vi "stopVILV2G.vi"(10 "Mode":enum16{"Init", "Get", "Set"}(ring), 11 "Stop IN":bool) -> (2 "Skipped?":bool=TRUE, 3 "Stop OUT":bool)   [LabVIEW 2010]
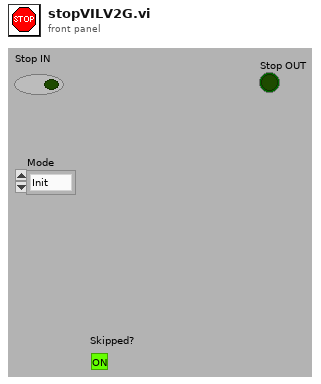
[diagram p1: front panel]
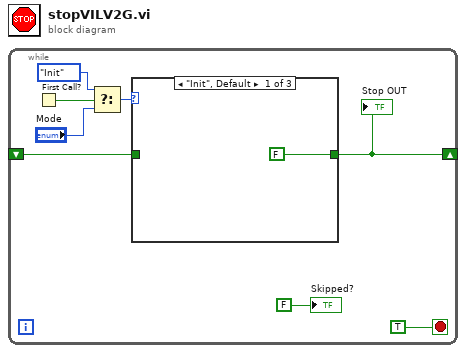
[diagram p0: block diagram]
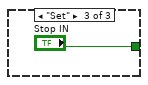
[diagram p3: hidden frame]
diagram:
  n1 = while {
    shift-right: [w6] -> _
    shift-left: _ -> [w5]
    stop <- TRUE stop-if-true
    n2 = First Call?() -> (First Call?: T/F=w3:bool)
    n3 = Select(t=enum16{"Init", "Get", "Set"}."Init" ("Mode"), s=w3, f="Mode") -> (s? t:f=w1:enum16{"Init", "Get", "Set"})
    n4 = case shown="\"Init\", Default" w1 {
      tunnel: [FALSE w10 "Stop IN"] -> w6
      tunnel: w5 -> [_ w10 _]
      frame "Init", Default {
      }
      frame "Get" {
      }
      frame "Set" {
      }
    }
    "Stop OUT" <- w6
    "Skipped?" <- FALSE ("Skipped?")
  }
